vi "Test Device by Resource.vi"() -> ()   [LabVIEW 2020]
uses:
  Builds/picoG/ppl/PicoG-Core.lvlibp/PicoG-Processor/PicoG-Core/Device/Device Info.ctl
  Builds/picoG/ppl/PicoG-Core.lvlibp/PicoG-Processor/PicoG-Core/VisaResource/VisaResource.lvclass
  Builds/picoG/ppl/PicoG-Core.lvlibp/PicoG-Processor/PicoG-Core/DeviceManager/DeviceManager.lvclass
  Builds/picoG/ppl/PicoG-Core.lvlibp/PicoG-Processor/PicoG-Core/Device/Device.lvclass
  C:/dev/Vireo/PicoG/Builds/picoG/ppl/PicoG-Core.lvlibp/PicoG-Processor/PicoG-Core/DeployResource/DeployResource.lvclass
panel:
  out "Devices":T1[](array[typedef])
  in  "Resource":refnum<visa-resource-name>
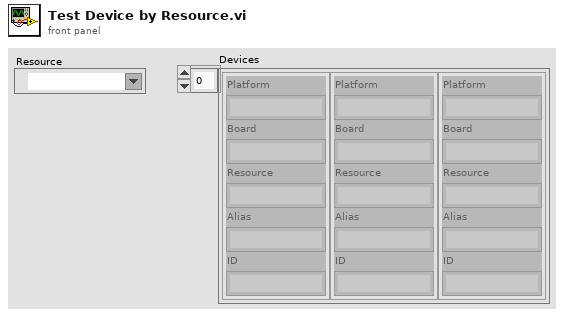
[diagram p1: front panel]
types:
  T1 = typedef "PicoG-Core.lvlibp/Device.lvclass/Device Info.ctl" = cluster{"Platform":string, "Board":string, "Resource":string, "Alias":string, "ID":string}
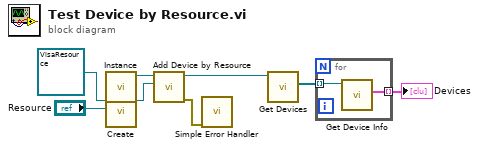
[diagram p0: block diagram]
diagram:
  n1 = call "Instance.vi"() -> ("Device Manager"=w6:refnum<class "DeviceManager.lvclass">)  [unwired: 10 in, 1 out]
  n2 = call-dynamic "Create.vi"("Resource"="Resource", "VisaResource in"=refnum<class "VisaResource.lvclass"> refnum) -> ("VisaResource out"=w5:refnum<class "VisaResource.lvclass">)  [unwired: 8 in, 1 out]
  n3 = call "Add Device by Resource.vi"("Resource"=w5, "DeviceManager in"=w6) -> ("error out"=w4:errorcluster, "DeviceManager out"=w3:refnum<class "DeviceManager.lvclass">)  [unwired: 7 in, 1 out]
  n4 = call <vilib>:"Simple Error Handler.vi"("error in (no error)"=w4) -> ()  [unwired: 4 in, 5 out]
  n5 = call "Get Devices.vi"("DeviceManager in"=w3) -> ("Devices"=w2:refnum<class "Device.lvclass">[])  [unwired: 8 in, 2 out]
  n6 = for {
    tunnel: w2 -> [w10] mode=indexing
    tunnel: [w9] -> w1 mode=indexing
    n7 = call "Get Device Info.vi"("Device in"=w10) -> ("Device Info"=w9:T1)  [unwired: 8 in, 2 out]
  }
  "Devices" <- w1
